vi "move complete.vi"(8 "error in (no error)":errorcluster caption="错误输入（无错误）", 9 "minimal error":dbl, 10 "Position":dbl[](array[numeric]), 11 "target position":dbl) -> (0 "error out":errorcluster caption="错误输出", 2 "move complete":bool, 3 "position output":dbl)   [LabVIEW 2017]
doc: "本VI 是仪器控制中的一个小程序，用于判断电机已经移动完毕，然后就停止刷新位置信息，该VI就是为了灵活地更新位置信息，避免浪费时间又尽量保证位置信息是准确的。具体做法就是当目标值和当前坐标值相差在最小误差之内时，停止更新坐标的循环。"
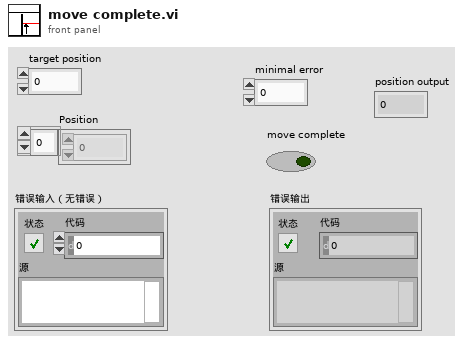
[diagram p1: front panel]
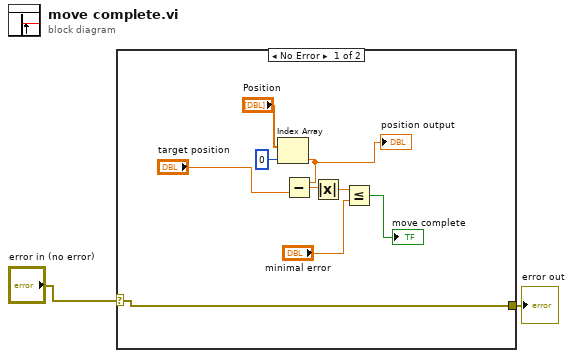
[diagram p0: block diagram]
diagram:
  n1 = case shown="No Error" "error in (no error)" {
    selector: "error in (no error)" -> [w3 w12]
    tunnel: [w3 w12] -> w1
    frame No Error {
      n2 = Index Array(array="Position", index=0 ("索引")) -> (element=w4:dbl)
      "position output" <- w4
      n3 = Subtract(x=w4, y="target position") -> (x-y=w11:dbl)
      n4 = Absolute Value(x=w11) -> (abs(x)=w7:dbl)
      n5 = Less Or Equal?(x=w7, y="minimal error") -> (x <= y?=→"move complete":bool)
    }
    frame Error {
    }
  }
  "error out" <- w1
